vi "adasda.vi"(6 "cos amp":dbl=1.0, 7 "Puntkide arv":i32=600, 8 "error in (no error)":errorcluster, 9 "sin amp":dbl=1.0, 10 "cos sagedus":dbl=1.0, 11 "sin sagedus":dbl=1.0) -> (0 "error out":errorcluster, 3 "appended array":cluster{i32, i32, dbl[]}[](array[cluster]))   [LabVIEW 2020]
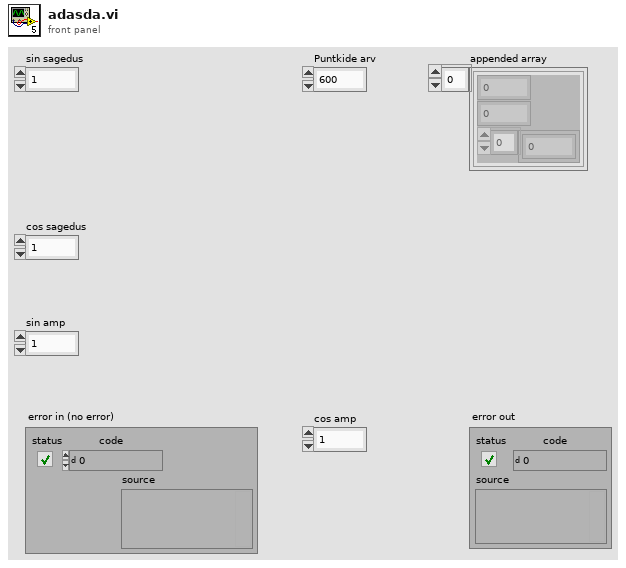
[diagram p1: front panel]
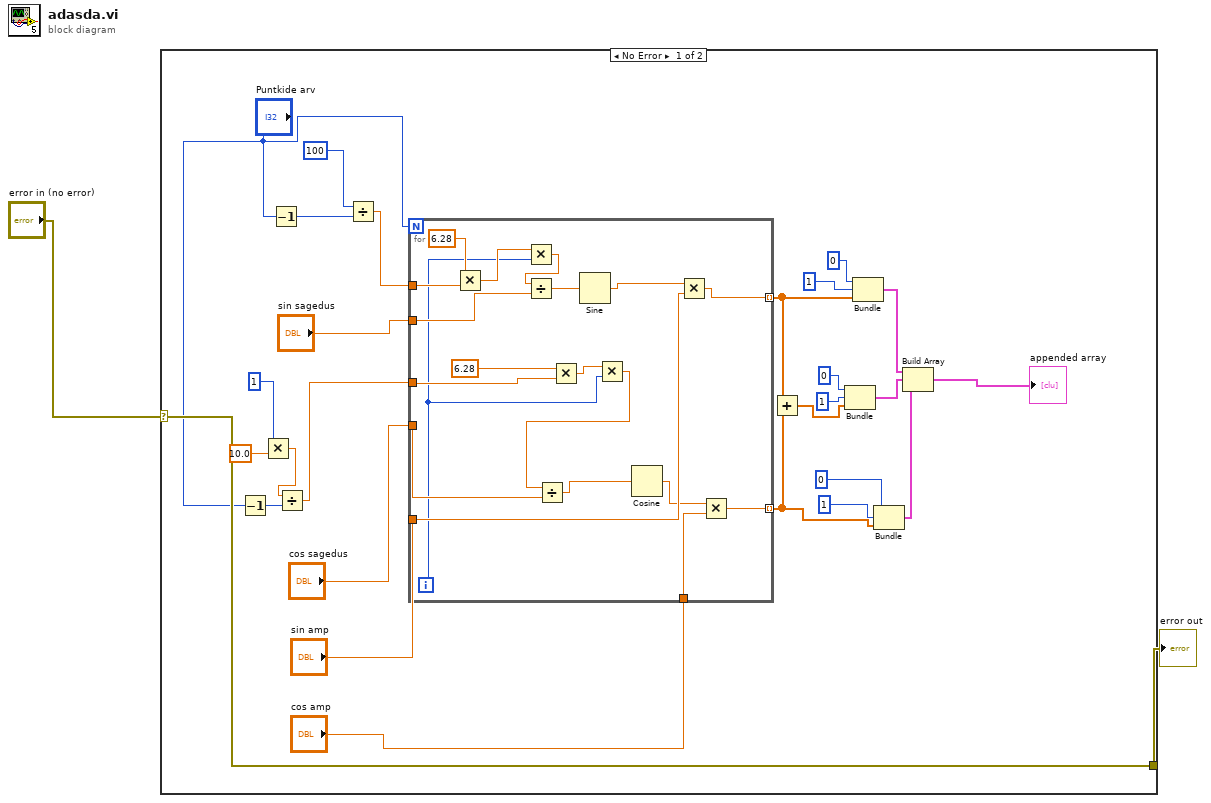
[diagram p0: block diagram]
diagram:
  n1 = case shown="No Error" "error in (no error)" {
    selector: "error in (no error)" -> [w29 w49]
    tunnel: [w29 w49] -> w2
    frame No Error {
      n2 = Decrement(x="Puntkide arv") -> (x-1=w10:i32)
      n3 = Multiply(x=1, y=10.0) -> (x*y=w4:dbl)
      n4 = Decrement(x="Puntkide arv") -> (x-1=w12:i32)
      n5 = Divide(x=w4, y=w10) -> (x/y=w7:dbl)
      n6 = Divide(x=100, y=w12) -> (x/y=w8:dbl)
      n7 = for {
        N: "Puntkide arv" -> [_]
        tunnel: "sin sagedus" -> [w48]
        tunnel: "cos sagedus" -> [w47]
        tunnel: "sin amp" -> [w44]
        tunnel: "cos amp" -> [w43]
        tunnel: [w40] -> w18 mode=indexing
        tunnel: [w39] -> w20 mode=indexing
        tunnel: w8 -> [w38]
        tunnel: w7 -> [w34]
        i -> [w31]
        n8 = Multiply(x=6.28, y=w38) -> (x*y=w36:dbl)
        n9 = Multiply(x=w36, y=w31) -> (x*y=w35:dbl)
        n10 = Divide(x=w35, y=w48) -> (x/y=w45:dbl)
        n11 = Multiply(x=6.28, y=w34) -> (x*y=w32:dbl)
        n12 = Sine(x=w45) -> (sin(x)=w42:dbl)
        n13 = Multiply(x=w32, y=w31) -> (x*y=w30:dbl)
        n14 = Divide(x=w30, y=w47) -> (x/y=w46:dbl)
        n15 = Cosine(x=w46) -> (cos(x)=w41:dbl)
        n16 = Multiply(x=w42, y=w44) -> (x*y=w39:dbl)
        n17 = Multiply(x=w41, y=w43) -> (x*y=w40:dbl)
      }
      n18 = Add(x=w20, y=w18) -> (x+y=w19:dbl[])
      n19 = Bundle(0, 1, w19) -> (w14:cluster{i32, i32, dbl[]})  [unwired: 1 in]
      n20 = Bundle(0, 1, w20) -> (w15:cluster{i32, i32, dbl[]})  [unwired: 1 in]
      n21 = Bundle(0, 1, w18) -> (w13:cluster{i32, i32, dbl[]})  [unwired: 1 in]
      n22 = Build Array(w15, w14, w13) -> (→"appended array":cluster{i32, i32, dbl[]}[])
    }
    frame Error {
    }
  }
  "error out" <- w2
